vi "Setup V0.80.vi"(6 "Control Parameters Input":T1={"Grating Density"=enum."1200", "Offset"=0.0, "Save All Data in ONE file"=FALSE, "Auto Save Data"=FALSE, "Most recent saved file"=path "erererere", "Filename Prefix"="MyData", "Extension"=4, "Suffix"="", "Current Path"=path "/DATA"} {"Extension" items=["DOS field", "\".001\",\".002\", ...", "001 (No dot)", "\".A\",\".B\", ...", "±Field", "pField nField", "Temperature", "User Defined"]; "Offset" format="%.2f"}, 7 "TempControl Input":bool[](array[boolean])=[TRUE, FALSE, FALSE, FALSE], 8 "Parameters#2 input":T2={"MaxBufferSize"=2, "Mag GPIB Address"=5, "Max Current (kA)"=36.0, "LTC-GPIB Address"="", "Temp Tolerance"=1.0} {"Temp Tolerance" format="%.2f"; "Max Current (kA)" format="%.2f"}, 9 "Parameters Input":T3={"Magnetic Field"=0.0, "Temperature"=0.0, "Exposure Time"=0.0, "Mag ID string"="", "User Name"="Albert Einstein", "Comments"="", "SaveComments?"=1, "X-Axis Unit"=1, "Delimiter"=0, "File Format"=0, "Sample Name"="Sample1"} {"File Format" items=["Macintosh (EOL: CR)", "Unix (EOL: LF)", "DOS/Windows (EOL: CR+LF)"]; "Delimiter" items=["TAB", "COMMA", "SPACE"]; "X-Axis Unit" items=["Point #", "nm", "eV", "meV", "cm-1"]; "SaveComments?" items=["Bare data only", "Saved in the Header Area", "Saved as a Parameter File"]; "Exposure Time" format="%.2f"; "Temperature" format="%.2f"; "Magnetic Field" format="%.2f"}) -> (0 "Control Parameters output":T1={"Grating Density"=enum."1200", "Offset"=0.0, "Save All Data in ONE file"=FALSE, "Auto Save Data"=FALSE, "Most recent saved file"=path "erererere", "Filename Prefix"="MyData", "Extension"=4, "Suffix"="", "Current Path"=path "/DATA"} {"Extension" items=["DOS field", "\".001\",\".002\", ...", "001 (No dot)", "\".A\",\".B\", ...", "±Field", "pField nField", "Temperature", "User Defined"]; "Offset" format="%.2f"}, 1 "Parameters#2":T2={"MaxBufferSize"=2, "Mag GPIB Address"=5, "Max Current (kA)"=36.0, "LTC-GPIB Address"="", "Temp Tolerance"=1.0} {"Temp Tolerance" format="%.2f"; "Max Current (kA)" format="%.2f"}, 2 "TempControl":bool[](array[boolean])=[TRUE, FALSE, FALSE, FALSE], 3 "Parameters output":T3={"Magnetic Field"=0.0, "Temperature"=0.0, "Exposure Time"=0.0, "Mag ID string"="None", "User Name"="", "Comments"="", "SaveComments?"=1, "X-Axis Unit"=1, "Delimiter"=0, "File Format"=0, "Sample Name"="Sample1"} {"File Format" items=["Macintosh (EOL: CR)", "Unix (EOL: LF)", "DOS/Windows (EOL: CR+LF)"]; "Delimiter" items=["TAB", "COMMA", "SPACE"]; "X-Axis Unit" items=["Point #", "nm", "eV", "meV", "cm-1"]; "SaveComments?" items=["Bare data only", "Saved in the Header Area", "Saved as a Parameter File"]; "Exposure Time" format="%.2f"; "Temperature" format="%.2f"; "Magnetic Field" format="%.2f"}, 4 "McP off":bool=TRUE caption="McP on? output", 5 "CCD off":bool=TRUE caption="CCD on? output")   [LabVIEW 2019]
uses:
  Parameters#1.ctl
  Parameters#2.ctl
  Parameters#Control.ctl
  Globals and TypeDefs/Global Varibal Control.vi
  ExperimentLogGlobal.vi
panel:
  in  "Maximum BufferSize":u8=50 min=1 step=1
  in  "OpenUserProfile":bool
  out "Clock copy":string="1:26:45 AM"
  out "Clock":string="1:26:45 AM"
  in  "McP on?":bool=TRUE caption="Off"
  in  "CCD on?":bool=TRUE caption="Off"
  out "CCD GPIB Address":u8=1 min=1 max=30
  in  "CCD LineSet?":bool caption="The CCD has NOT been initialized yet."
  in  "ChangeCounterPos?":bool
  in  "?":bool
  in  "LTC20 Cal Table?":bool
  in  "Hide?":bool
  out "GPIB Status":string
  in  "BusScan?":bool
  in  "Calibration":bool
  in  "X-Axis Unit":u16(ring)=1 items=["Point #", "nanometer (nm)", "electron volt (eV)", "Milli eV (meV)", "Wavenumber (cm-1)"]
  in  "SaveComments?":u16(ring)=1 items=["Bare data only", "Saved in the Header Area", "Saved as a Parameter File"]
  in  "Delimiter":u16(ring) items=["TAB", "COMMA", "SPACE"]
  in  "File Format":u16(ring) items=["Macintosh (EOL: CR)", "Unix (EOL: LF)", "DOS/Windows (EOL: CR+LF)"]
  in  "Max Current (kA)":dbl=36.0 caption="Maximum Current (kA)" format="%.2f"
  in  "User Name":string
  in  "Temp Tolerance":dbl=1.0 caption="Temperature Tolerance (if applicable)" format="%.2f"
  in  "LTC-GPIB Address":refnum<visa-resource-name> caption="GPIB Address"
  in  "Auto\nAdvance?":bool
  in  "Magneto\nCorrection?":bool
  in  "Mode:\nControl?":bool caption="Monitor"
  in  "LTC-20\nexist?":bool
  in  "McP init?":bool caption="The spectrometer has NOT been initialized yet."
  in  "SaveUserProfile":bool
  in  "Sample Name":string="Sample1"
  # "User Profile Panel"
  # "Magnet Control Panel"
  # "The Modem Port is reserved."
  # "Conductus LTC-20 Panel"
  # "Yes\n\nNo"
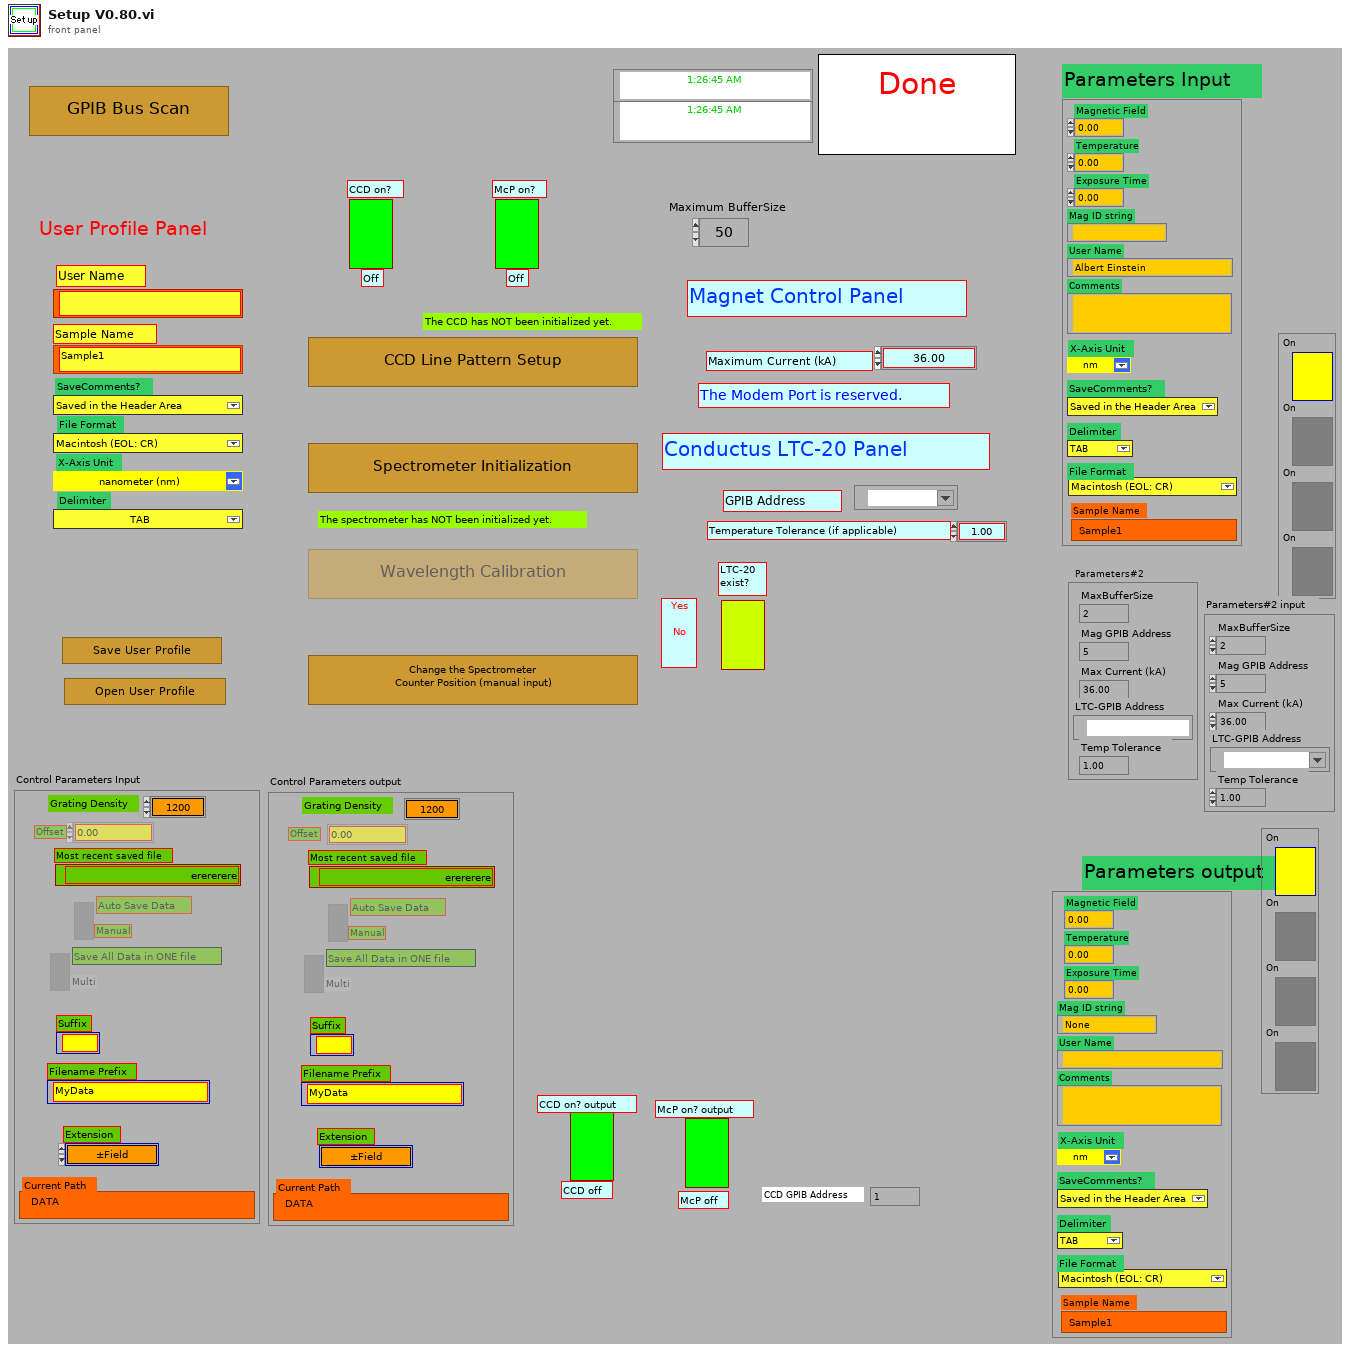
[diagram p1: front panel]
types:
  T1 = typedef "Parameters#Control.ctl" = cluster{"Grating Density":enum16{"150", "300", "600", "1200", "1800"}, "Offset":dbl, "Save All Data in ONE file":bool, "Auto Save Data":bool, "Most recent saved file":path, "Filename Prefix":string, "Extension":u16, "Suffix":string, "Current Path":path}
  T2 = typedef "Parameters#2.ctl" = cluster{"MaxBufferSize":i32, "Mag GPIB Address":i32, "Max Current (kA)":dbl, "LTC-GPIB Address":refnum<visa-resource-name>, "Temp Tolerance":dbl}
  T3 = typedef "Parameters#1.ctl" = cluster{"Magnetic Field":dbl, "Temperature":dbl, "Exposure Time":dbl, "Mag ID string":string, "User Name":string, "Comments":string, "SaveComments?":u16, "X-Axis Unit":u16, "Delimiter":u16, "File Format":u16, "Sample Name":string}
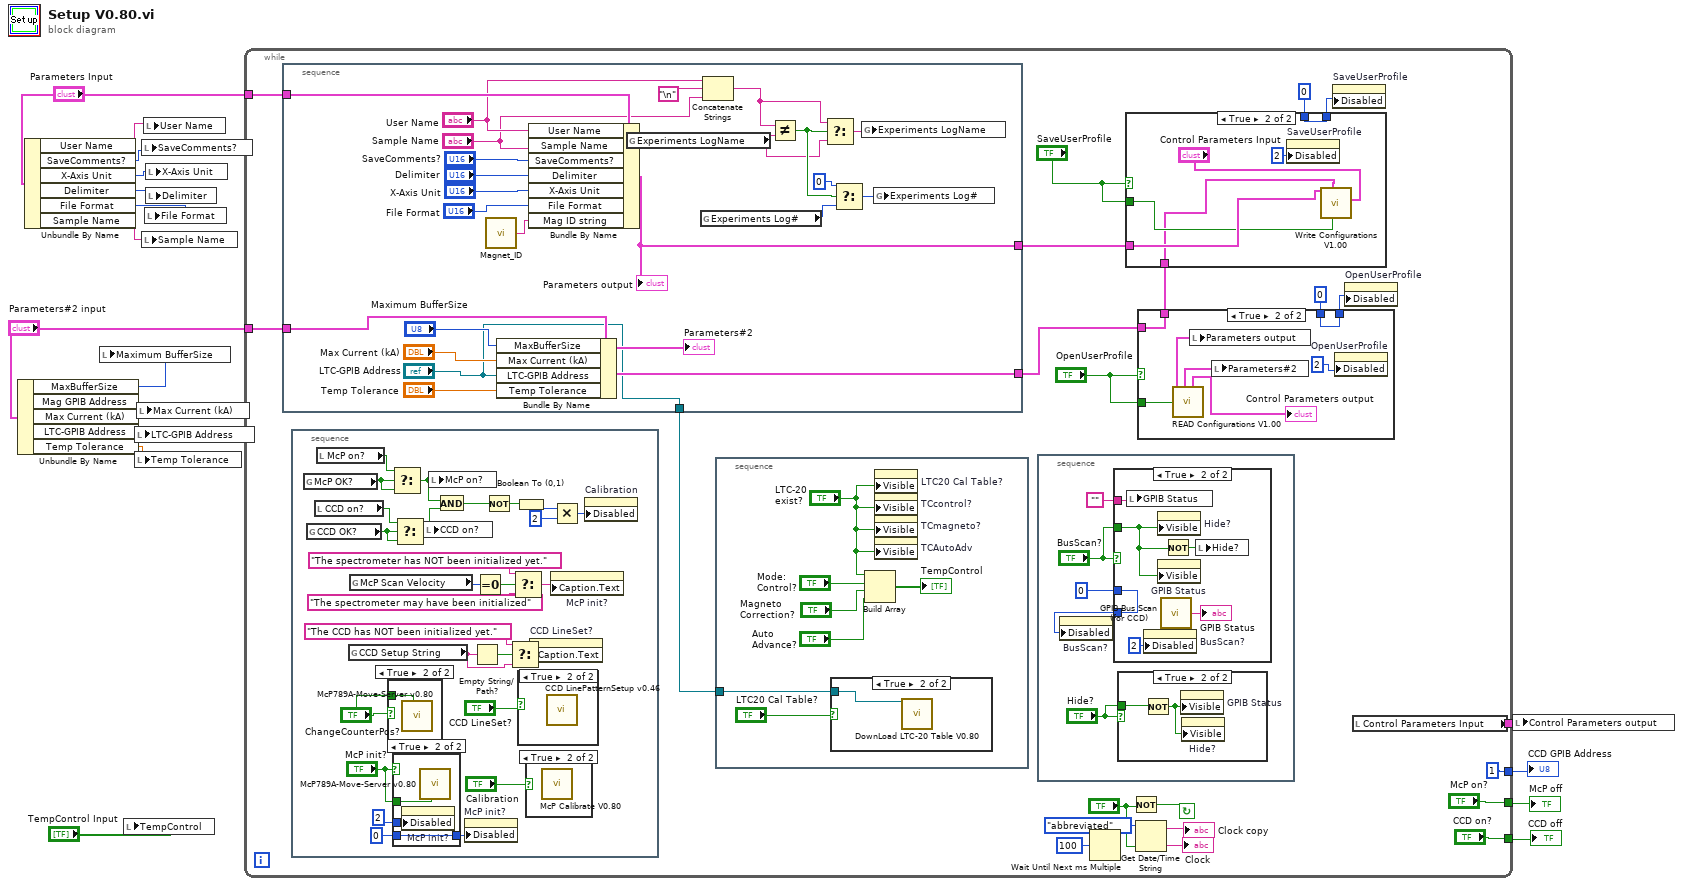
[diagram p0: block diagram]
diagram:
  n1 = Unbundle By Name("Parameters#2 input") -> ("MaxBufferSize"=w2:i32, "Max Current (kA)"=w8:dbl, "LTC-GPIB Address"=w7:refnum<visa-resource-name>, "Temp Tolerance"=w6:dbl)  [unwired: 1 out]
  n2 = Unbundle By Name("Parameters Input") -> ("User Name"=w10:string, "SaveComments?"=w11:u16, "X-Axis Unit"=w12:u16, "Delimiter"=w13:u16, "File Format"=w14:u16, "Sample Name"=w15:string)
  n3 = local write "Maximum BufferSize"(w2) -> ()
  n4 = local write "TempControl"("TempControl Input") -> ()
  n5 = local write "LTC-GPIB Address"(w7) -> ()
  n6 = local write "Temp Tolerance"(w6) -> ()
  n7 = local write "Max Current (kA)"(w8) -> ()
  n8 = local write "SaveComments?"(w11) -> ()
  n9 = local write "Sample Name"(w15) -> ()
  n10 = local write "User Name"(w10) -> ()
  n11 = local write "File Format"(w14) -> ()
  n12 = local write "X-Axis Unit"(w12) -> ()
  n13 = local write "Delimiter"(w13) -> ()
  n14 = while {
    tunnel: [w18] -> w1
    tunnel: ["CCD on?"] -> w3
    tunnel: ["McP on?"] -> w4
    tunnel: "Parameters#2 input" -> [w35]
    tunnel: "Parameters Input" -> [w36]
    tunnel: [1] -> w17
    stop <- w39 continue-if-true
    n15 = stacked-sequence {
      tunnel: w36 -> [w115]
      tunnel: w35 -> [w101]
      tunnel: ["LTC-GPIB Address"] -> w28
      tunnel: [w103] -> w25
      tunnel: [w102] -> w24
      frame #0 {
        n16 = call "Magnet_ID.vi"() -> ("Cell"=w97:string)
        n17 = Bundle By Name(cluster=w101, "MaxBufferSize"="Maximum BufferSize", "Max Current (kA)"="Max Current (kA)", "LTC-GPIB Address"="LTC-GPIB Address", "Temp Tolerance"="Temp Tolerance") -> (w102:T2)
        "Parameters#2" <- w102
        n18 = Bundle By Name(cluster=w115, "User Name"="User Name", "Sample Name"="Sample Name", "SaveComments?"="SaveComments?", "Delimiter"="Delimiter", "X-Axis Unit"="X-Axis Unit", "File Format"="File Format", "Mag ID string"=w97) -> (w103:T3)
        "Parameters output" <- w103
        n19 = global read "ExperimentLogGlobal.vi" "Experiments LogName"() -> (w105:string)
        n20 = global read "ExperimentLogGlobal.vi" "Experiments Log#"() -> (w106:u32)
        n21 = Concatenate Strings("User Name", "\n", "Sample Name") -> (w110:string)
        n22 = Not Equal?(x=w110, y=w105) -> (x != y?=w109:bool)
        n23 = Select(t=w110, s=w109, f=w105) -> (s? t:f=w104:string)
        n24 = Select(t=0, s=w109, f=w106) -> (s? t:f=w107:u32)
        n25 = global write "ExperimentLogGlobal.vi" "Experiments LogName"(w104) -> ()
        n26 = global write "ExperimentLogGlobal.vi" "Experiments Log#"(w107) -> ()
      }
    }
    n27 = stacked-sequence {
      frame #0 {
        n28 = global read "Global Varibal Control.vi" "McP OK?"() -> (w70:bool)
        n29 = global read "Global Varibal Control.vi" "CCD OK?"() -> (w68:bool)
        n30 = local read "CCD on?"() -> (w69:bool)
        n31 = local read "McP on?"() -> (w71:bool)
        n32 = global read "Global Varibal Control.vi" "CCD Setup String"() -> (w73:string)
        n33 = global read "Global Varibal Control.vi" "McP Scan Velocity"() -> (w80:i32)
        n34 = case shown="True" "ChangeCounterPos?" {
          tunnel: "ChangeCounterPos?" -> [_ w83]
          frame False {
          }
          frame True {
            n35 = call "McP789A-Move-Server v0.80.vi"("Change Counter Position Manually"=w83) -> ()  [unwired: 5 in, 5 out]
          }
        }
        n36 = Select(t=w71, s=w70, f=w70) -> (s? t:f=w67:bool)
        n37 = case shown="True" "McP init?" {
          tunnel: "McP init?" -> [_ w87]
          tunnel: i16 2 ("y") -> [_ w86]
          tunnel: i16 0 ("y") -> [w84 w85]
          tunnel: [w84 w85] -> w56
          frame False {
          }
          frame True {
            n38 = property on="McP init?" class="Bool"("Disabled"=w86) -> ()  [unwired: 2 in, 2 out]
            n39 = call "McP789A-Move-Server v0.80.vi"("Initializing MCP"=w87) -> ()  [unwired: 5 in, 5 out]
          }
        }
        n40 = Select(t=w69, s=w68, f=w68) -> (s? t:f=w66:bool)
        n41 = local write "CCD on?"(w66) -> ()
        n42 = local write "McP on?"(w67) -> ()
        n43 = And(x=w67, y=w66) -> (x .and. y?=w62:bool)
        n44 = property on="McP init?" class="Bool"("Disabled"=w56) -> ()  [unwired: 2 in, 2 out]
        n45 = Empty String/Path?(string/path=w73) -> (empty?=w75:bool)
        n46 = Equal To 0?(x=w80) -> (x = 0?=w79:bool)
        n47 = Not(x=w62) -> (.not. x?=w65:bool)
        n48 = Select(t="The CCD has NOT been initialized yet.", s=w75, f=w73) -> (s? t:f=w72:string)
        n49 = Select(t="The spectrometer has NOT been initialized yet.", s=w79, f="The spectrometer may have been initialized") -> (s? t:f=w78:string)
        n50 = Boolean To (0,1)(Boolean=w65) -> (0, 1=w64:i16)
        n51 = case shown="True" "CCD LineSet?" {
          frame False {
          }
          frame True {
            n52 = call "CCD LinePatternSetup v0.46.vi"() -> ()  [unwired: 9 in, 2 out]
          }
        }
        n53 = case shown="True" "Calibration" {
          frame False {
          }
          frame True {
            n54 = call "McP Calibrate V0.80.vi"() -> ()  [unwired: 1 in]
          }
        }
        n55 = property on="CCD LineSet?" class="Bool"("Caption.Text"=w72) -> ()  [unwired: 2 in, 2 out]
        n56 = property on="McP init?" class="Bool"("Caption.Text"=w78) -> ()  [unwired: 2 in, 2 out]
        n57 = Multiply(x=w64, y=i16 2) -> (x*y=w61:i16)
        n58 = property on="Calibration" class="Bool"("Disabled"=w61) -> ()  [unwired: 2 in, 2 out]
      }
    }
    n59 = stacked-sequence {
      tunnel: w28 -> [w88]
      frame #0 {
        n60 = case shown="True" "LTC20 Cal Table?" {
          tunnel: w88 -> [_ w95]
          frame False {
          }
          frame True {
            n61 = call "DownLoad LTC-20 Table V0.80.vi"("LTC-20 GPIB"=w95) -> ()  [unwired: 16 in, 3 out]
          }
        }
        n62 = Build Array("LTC-20\nexist?", "Mode:\nControl?", "Magneto\nCorrection?", "Auto\nAdvance?") -> (→"TempControl":bool[])
        n63 = property on="LTC20 Cal Table?" class="Bool"("Visible"="LTC-20\nexist?") -> ()  [unwired: 2 in, 2 out]
        n64 = property on="TCcontrol?" class="Bool (strict)"("Visible"="LTC-20\nexist?") -> ()  [unwired: 2 in, 2 out]
        n65 = property on="TCmagneto?" class="Bool (strict)"("Visible"="LTC-20\nexist?") -> ()  [unwired: 2 in, 2 out]
        n66 = property on="TCAutoAdv" class="Bool (strict)"("Visible"="LTC-20\nexist?") -> ()  [unwired: 2 in, 2 out]
      }
    }
    n67 = stacked-sequence {
      frame #0 {
        n68 = case shown="True" "BusScan?" {
          tunnel: "" -> [_ w131]
          tunnel: "BusScan?" -> [_ w129]
          tunnel: [w126 w127] -> w119
          tunnel: u8 0 ("Write Attribute") -> [w126 w127]
          frame False {
          }
          frame True {
            n69 = local write "GPIB Status"(w131) -> ()
            n70 = property on="BusScan?" class="Bool"("Disabled"=u8 2 ("Write Attribute")) -> ()  [unwired: 2 in, 2 out]
            n71 = property on="Hide?" class="Bool (strict)"("Visible"=w129) -> ()  [unwired: 2 in, 2 out]
            n72 = property on="GPIB Status" class="Str"("Visible"=w129) -> ()  [unwired: 2 in, 2 out]
            n73 = call "GPIB Bus Scan (for CCD).vi"() -> (0:→"GPIB Status":string)  [unwired: 1 in]
            n74 = Not(x=w129) -> (.not. x?=w130:bool)
            n75 = local write "Hide?"(w130) -> ()
          }
        }
        n76 = property on="BusScan?" class="Bool"("Disabled"=w119) -> ()  [unwired: 2 in, 2 out]
        n77 = case shown="True" "Hide?" {
          tunnel: "Hide?" -> [_ w125]
          frame False {
          }
          frame True {
            n78 = Not(x=w125) -> (.not. x?=w124:bool)
            n79 = property on="GPIB Status" class="Str"("Visible"=w124) -> ()  [unwired: 2 in, 2 out]
            n80 = property on="Hide?" class="Bool (strict)"("Visible"=w124) -> ()  [unwired: 2 in, 2 out]
          }
        }
      }
    }
    n81 = Wait Until Next ms Multiple(millisecond multiple=u32 100) -> ()  [unwired: 1 out]
    n82 = Not(x="?") -> (.not. x?=w39:bool)
    n83 = Get Date/Time String(date format (0)=enum16{"short", "long", "abbreviated"}."abbreviated", want seconds? (F)="?") -> (date string=→"Clock copy":string, time string=→"Clock":string)  [unwired: 1 in]
    n84 = case shown="True" "OpenUserProfile" {
      tunnel: "OpenUserProfile" -> [_ w45]
      tunnel: [w41 w44] -> w23
      tunnel: w24 -> [w41 w44]
      tunnel: [w40 w43] -> w20
      tunnel: u8 0 ("Write Attribute") -> [w40 w43]
      frame False {
      }
      frame True {
        n85 = call "READ Configurations V1.00.vi"("OpenParameters(T)orDataBuffers(F)"=w45) -> ("Parameters"=w47:T3, "Parameters#2"=w46:T2, "Control Parameters"=→"Control Parameters output":T1)  [unwired: 2 in, 4 out]
        n86 = local write "Parameters output"(w47) -> ()
        n87 = local write "Parameters#2"(w46) -> ()
        n88 = property on="OpenUserProfile" class="Bool"("Disabled"=u8 2 ("Write Attribute")) -> ()  [unwired: 2 in, 2 out]
      }
    }
    n89 = case shown="True" "SaveUserProfile" {
      tunnel: "SaveUserProfile" -> [_ w53]
      tunnel: w25 -> [_ w54]
      tunnel: w23 -> [_ w52]
      tunnel: [w49 w50] -> w22
      tunnel: u8 0 ("Write Attribute") -> [w49 w50]
      frame False {
      }
      frame True {
        n90 = property on="SaveUserProfile" class="Bool"("Disabled"=u8 2 ("Write Attribute")) -> ()  [unwired: 2 in, 2 out]
        n91 = call "Write Configurations V1.00.vi"("Control Parameters"="Control Parameters Input", "SaveParameters(T)/DataBuffer(F)?"=w53, "Parameters#2"=w52, "Parameters"=w54) -> ()  [unwired: 6 in, 1 out]
      }
    }
    n92 = property on="SaveUserProfile" class="Bool"("Disabled"=w22) -> ()  [unwired: 2 in, 2 out]
    n93 = property on="OpenUserProfile" class="Bool"("Disabled"=w20) -> ()  [unwired: 2 in, 2 out]
    n94 = local read "Control Parameters Input"() -> (w18:T1)
  }
  "CCD GPIB Address" <- w17
  "CCD off" <- w3
  "McP off" <- w4
  n95 = local write "Control Parameters output"(w1) -> ()
